vi "Actor Core.vi"(8 "error in":errorcluster, 11 "MainController in":refnum<class "MainController.lvclass">) -> (0 "error out":errorcluster, 3 "Actor out":refnum<class "Actor.lvclass">)   [LabVIEW 2012, in "Win8uiFramework.lvlib" / "MainController.lvclass"]
doc: "(<B>Filename</B>: Actor Framework.lvlib:Actor.lvclass:Actor Core.vi)\n\nReceives messages to the actor, reacts to them, and initiates any error handling that may shut the actor down.\n\nDescendant classes may override this VI to append parallel tasks for the actor to complete while it handles messages. Overrides use the Call Parent Method node."
uses:
  MainController.lvclass
  <vilib>/ActorFramework/Actor/Actor.lvclass
  <vilib>/ActorFramework/Time-Delayed Send Message/Time-Delay Override Options.ctl
  ViewableActor.lvclass/ViewableActor.ctl
  MainController.lvclass/MainController.ctl
  <vilib>/ActorFramework/Actor/Actor.lvclass/Actor.ctl
  <vilib>/ActorFramework/Message Enqueuer/Message Enqueuer.lvclass/Message Enqueuer.ctl
  ViewableActor.lvclass
  Display AppBar Msg.lvclass
  Hide AppBar Msg.lvclass
  Hide Charm Msg.lvclass/Hide Charm Msg.ctl
  Read Stop Event.vi
  Write Active SubPanel.vi
  Write Inactive SubPanel.vi
  Write AppBar Splitter.vi
  Write AppBar SubPanel.vi
  Write Charm Splitter.vi
  Write Charm SubPanel.vi
  Write UI VI Ref.vi
  Write Main Pane.vi
  Write Title Ref.vi
  <vilib>/ActorFramework/Message Enqueuer/Init from Existing Queue.vi
  <vilib>/ActorFramework/Message Enqueuer/Enqueue.vi
  <vilib>/ActorFramework/Message Priority Queue/Priority Enqueue.vi
  <vilib>/ActorFramework/Message Enqueuer/Message Enqueuer.lvclass
  <vilib>/ActorFramework/Stop Msg/Stop Msg.lvclass
  Resize Msg.lvclass
  Hide Charm Msg.lvclass
  Display Charm Msg.lvclass
  Win8uiFramework.lvlib
panel:
  out "Title":string="Application Title"
  out "Date":string
  out "Time":string
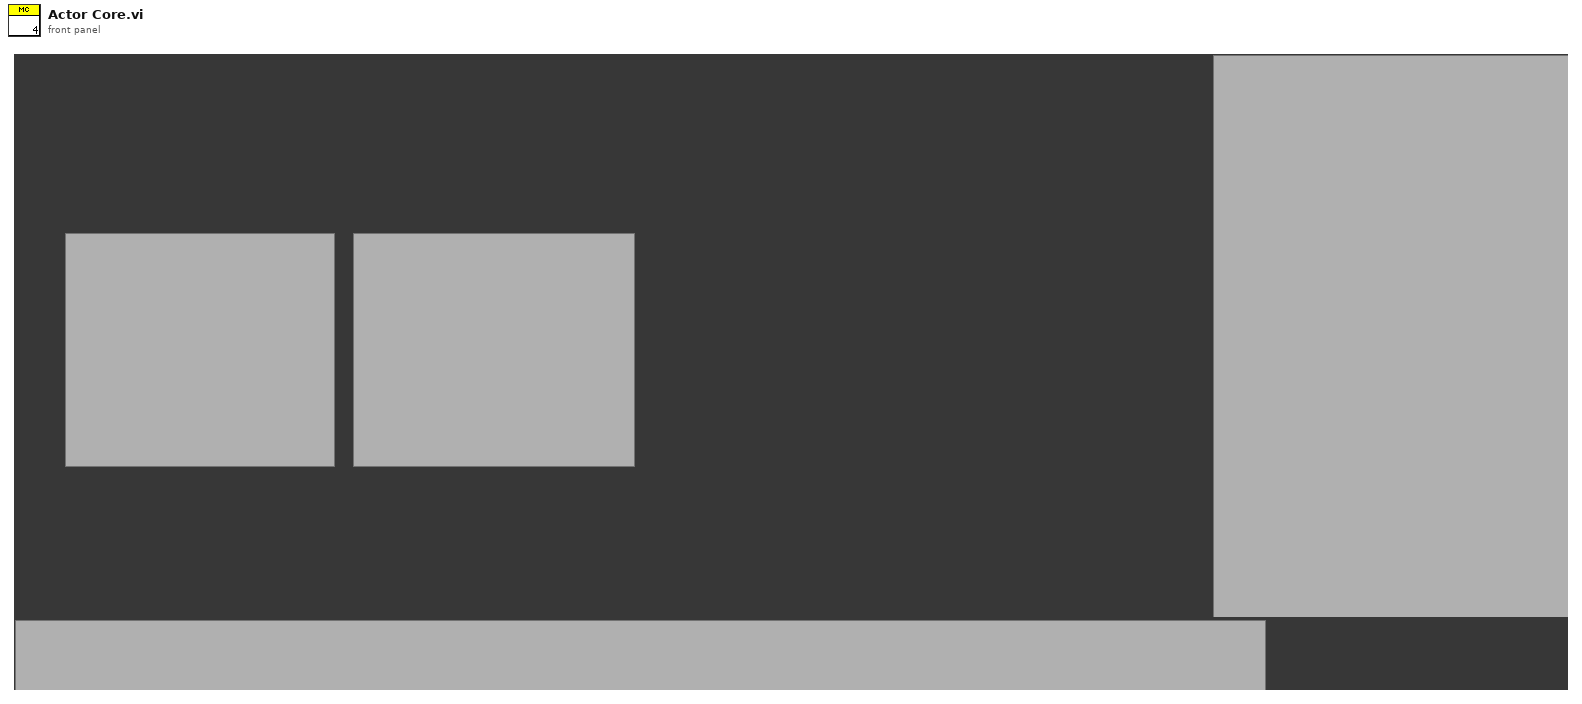
[diagram p1: front panel]
types:
  T1 = typedef "Time-Delay Override Options.ctl" = enum16{"Send next copy now", "Skip next scheduled copy", "Send next copy now and stop all further copies", "Stop all further copies"}
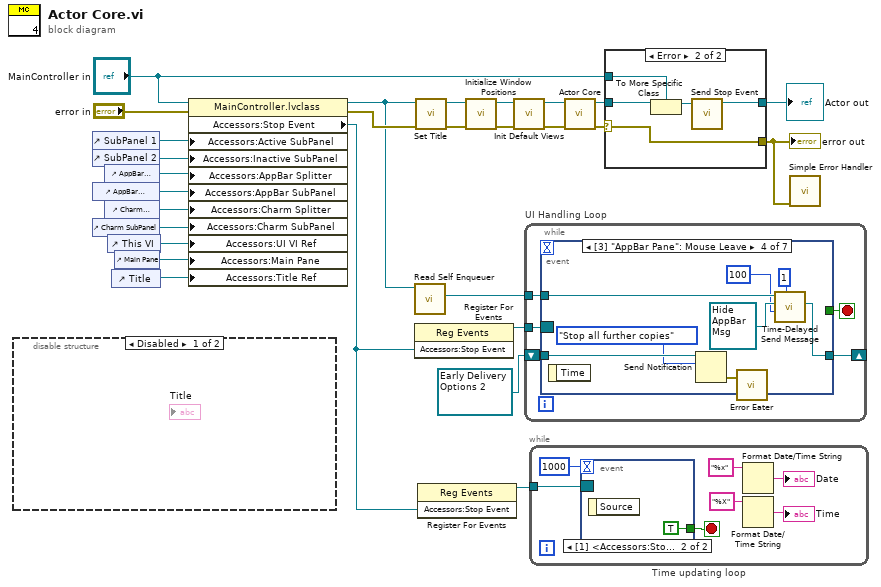
[diagram p0: block diagram]
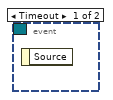
[diagram p3: hidden frame]
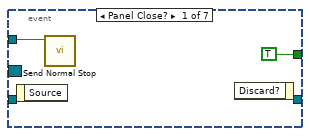
[diagram p4: hidden frame]
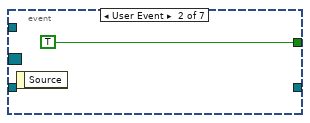
[diagram p5: hidden frame]
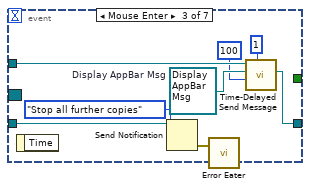
[diagram p6: hidden frame]
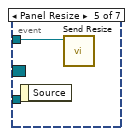
[diagram p7: hidden frame]
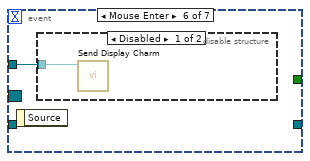
[diagram p8: hidden frame]
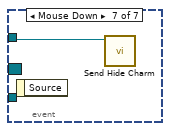
[diagram p10: hidden frame]
diagram:
  w1 = refnum<notifier> refnum items=["Send next copy now", "Skip next scheduled copy", "Send next copy now and stop all further copies", "Stop all further copies"] ("Delivery Notifier")
  n1 = disable-structure shown="Disabled" {
    frame Disabled {
    }
    frame Enabled {
    }
  }
  n2 = control-ref of="SubPanel 1"() -> (w16:refnum<vi>)
  n3 = control-ref of="SubPanel 2"() -> (w15:refnum<vi>)
  n4 = control-ref of="AppBar SubPanel"() -> (w18:refnum<vi>)
  n5 = control-ref of="Charm SubPanel"() -> (w19:refnum<vi>)
  n6 = control-ref of="AppBar Splitter"() -> (w13:refnum<vi>)
  n7 = control-ref of="Charm Splitter"() -> (w14:refnum<vi>)
  n8 = control-ref of="This VI"() -> (w17:refnum<vi>)
  n9 = control-ref of="Title"() -> (w7:refnum<vi>)
  n10 = control-ref of="Main Pane"() -> (w2:refnum<vi>)
  n11 = property class="MainController.lvclass"(reference="MainController in", error in="error in", "Accessors:Active SubPanel"=w16, "Accessors:Inactive SubPanel"=w15, "Accessors:AppBar Splitter"=w13, "Accessors:AppBar SubPanel"=w18, "Accessors:Charm Splitter"=w14, "Accessors:Charm SubPanel"=w19, "Accessors:UI VI Ref"=w17, "Accessors:Main Pane"=w2, "Accessors:Title Ref"=w7) -> (reference out=w3:refnum<class "MainController.lvclass">, error out=w4:errorcluster, "Accessors:Stop Event"=w21:refnum<user-event>)
  n12 = call <vilib>:"Read Self Enqueuer.vi"("Actor"=w3) -> ("Self Enqueuer"=w12:refnum<class "Message Enqueuer.lvclass">)  [unwired: 10 in]
  n13 = register-events(w21) -> (reference out=w28:refnum<event-registration>)  [unwired: 2 in, 1 out]
  n14 = call-dynamic "Set Title.vi"("error in (no error)"=w4, "MainController in"=w3) -> ("error out"=w5:errorcluster, "MainController out"=w6:refnum<class "MainController.lvclass">)  [unwired: 8 in]
  n15 = register-events(w21) -> (reference out=w20:refnum<event-registration>)  [unwired: 2 in, 1 out]
  n16 = call-dynamic "Initialize Window Positions.vi"("error in (no error)"=w5, "MainController in"=w6) -> ("error out"=w10:errorcluster, "MainController out"=w11:refnum<class "MainController.lvclass">)  [unwired: 8 in]
  n17 = call-dynamic "Init Default Views.vi"("error in (no error)"=w10, "MainController in"=w11) -> ("error out"=w8:errorcluster, "MainController out"=w9:refnum<class "MainController.lvclass">)  [unwired: 8 in]
  n18 = while "UI Handling Loop" {
    tunnel: w28 -> [w33]
    tunnel: w12 -> [w31]
    shift-right: [w30] -> _
    shift-left: w1 -> [w29]
    stop <- w32 stop-if-true
    n19 = event shown="[3] \"AppBar Pane\": Mouse Leave" {
      selector: w33 -> [_ _ _ _ _ _ _]
      dyn-events: _ -> [_ _ _ _ _ _ _]
      timeout: _ -> [_ _ _ _ _ _ _]
      tunnel: w31 -> [w35 _ w44 w51 w53 w54 w56]
      tunnel: [TRUE TRUE _ _ _ _ _] -> w32
      tunnel: [_ _ w41 w50 _ _ _] -> w30
      tunnel: w29 -> [_ _ w40 w48 _ _ _]
      event Panel Close? {
        n20 = event-data() -> ()  [unwired: 1 in, 1 out]
        n21 = call <vilib>:"Send Normal Stop.vi"("Message Enqueuer"=w35) -> ()  [unwired: 10 in, 1 out]
        n22 = event-data() -> ()  [unwired: 2 in, 1 out]
      }
      event User Event {
        n23 = event-data() -> ()  [unwired: 1 in, 1 out]
      }
      event Mouse Enter {
        w43 = refnum<class "Display AppBar Msg.lvclass"> refnum  # Display AppBar Msg
        n24 = event-data() -> ()  [unwired: 1 in, 1 out]
        n25 = Send Notification(notification=Time-Delay_Override_Options."Stop all further copies", notifier=w40) -> (error out=w39:errorcluster)  [unwired: 1 in, 1 out]
        n26 = call "Error Eater.vi"("error in (no error)"=w39) -> ()  [unwired: 2 in]
        n27 = call <vilib>:"Time-Delayed Send Message.vi"("# Copies (0 = infinite repeat)"=u32 1, "Milliseconds To Wait"=100, "Message"=w43, "Message Enqueuer"=w44) -> ("Delivery Notifier"=w41:refnum<notifier>)  [unwired: 6 in, 1 out]
      }
      event Mouse Leave {
        n28 = event-data() -> ()  [unwired: 1 in, 1 out]
        n29 = Send Notification(notification=Time-Delay_Override_Options."Stop all further copies", notifier=w48) -> (error out=w46:errorcluster)  [unwired: 1 in, 1 out]
        n30 = call "Error Eater.vi"("error in (no error)"=w46) -> ()  [unwired: 2 in]
        n31 = call <vilib>:"Time-Delayed Send Message.vi"("# Copies (0 = infinite repeat)"=u32 1, "Milliseconds To Wait"=100, "Message"=refnum<class "Hide AppBar Msg.lvclass"> refnum ("Object"), "Message Enqueuer"=w51) -> ("Delivery Notifier"=w50:refnum<notifier>)  [unwired: 6 in, 1 out]
      }
      event Panel Resize {
        n32 = event-data() -> ()  [unwired: 1 in, 1 out]
        n33 = call "Send Resize.vi"("Message Enqueuer"=w53) -> ()  [unwired: 9 in, 2 out]
      }
      event Mouse Enter {
        n34 = event-data() -> ()  [unwired: 1 in, 1 out]
        n35 = disable-structure shown="Disabled" {
          disable-tunnel: w54 -> [w55 _]
          frame Disabled {
            n36 = call "Send Display Charm.vi"("Message Enqueuer"=w55) -> ()  [unwired: 9 in, 2 out]
          }
          frame Enabled {
          }
        }
      }
      event Mouse Down {
        n37 = event-data() -> ()  [unwired: 1 in, 1 out]
        n38 = call "Send Hide Charm.vi"("Message Enqueuer"=w56) -> ()  [unwired: 9 in, 2 out]
      }
    }
  }
  n39 = while "Time updating loop" {
    tunnel: w20 -> [w63]
    stop <- w62 stop-if-true
    n40 = event shown="[1] <Accessors:Stop Event>: User Event" {
      selector: w63 -> [_ _]
      dyn-events: _ -> [_ _]
      timeout: 1000 -> [_ _]
      tunnel: [_ TRUE] -> w62
      event Timeout {
        n41 = event-data() -> ()  [unwired: 1 in, 1 out]
      }
      event User Event {
        n42 = event-data() -> ()  [unwired: 1 in, 1 out]
      }
    }
    n43 = Format Date/Time String(time format string (%c)="%x") -> (date/time string=→"Date":string)  [unwired: 2 in]
    n44 = Format Date/Time String(time format string (%c)="%X") -> (date/time string=→"Time":string)  [unwired: 2 in]
  }
  n45 = call-parent "Actor Core.vi"("error in"=w8, "Actor in"=w9) -> ("error out"=w26:errorcluster, "Actor out"=w25:refnum<class "Actor.lvclass">)  [unwired: 8 in]
  n46 = case shown="Error" w26 {
    selector: w26 -> [w65 w70]
    tunnel: w25 -> [w66 w69]
    tunnel: [w66 w71] -> w24
    tunnel: [w65 w70] -> w22
    tunnel: "MainController in" -> [_ w67]
    frame No Error {
    }
    frame Error {
      n47 = To More Specific Class(target class=w67, reference=w69) -> (specific class reference=w68:refnum<class "MainController.lvclass">)  [unwired: 1 in, 1 out]
      n48 = call-dynamic "Send Stop Event.vi"("ViewableActor in"=w68) -> ("ViewableActor out"=w71:refnum<class "MainController.lvclass">)  [unwired: 9 in, 1 out]
    }
  }
  "error out" <- w22
  "Actor out" <- w24
  n49 = call <vilib>:"Simple Error Handler.vi"("error in (no error)"=w22) -> ()  [unwired: 4 in, 5 out]
